vi "Graph_Get Attributes.vi"(8 "error in (no error)":errorcluster, 11 "reference in":refnum<class "Graph.lvclass">) -> (0 "error out":errorcluster, 1 "Graph DVR":refnum<data-value>, 2 "Graph Attributes":T1, 3 "reference out":refnum<class "Graph.lvclass">)   [LabVIEW 2017, in "Front Panel Publisher.lvlib" / "Graph.lvclass"]
uses:
  Graph.lvclass
  Attributes.ctl
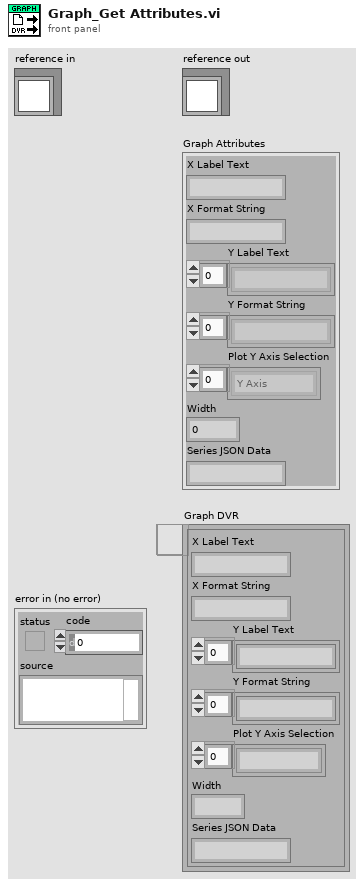
[diagram p1: front panel]
types:
  T1 = typedef "Front Panel Publisher.lvlib/Graph.lvclass/Attributes.ctl" = cluster{"X Label Text":string, "X Format String":string, "Y Label Text":string[], "Y Format String":string[], "Plot Y Axis Selection":enum16{"Y Axis", "Y2 Axis"}[], "Width":u32, "Series JSON Data":string}
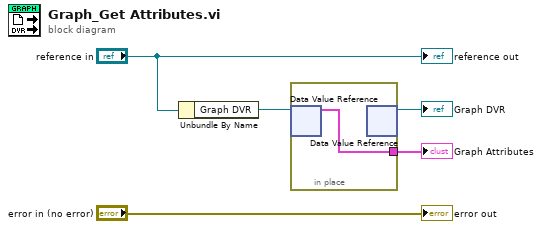
[diagram p0: block diagram]
diagram:
  n1 = Unbundle By Name("reference in") -> ("Graph DVR"=w3:refnum<data-value>)
  n2 = in-place {
    in-place-border: [w6] -> w2
    n3 = in-place-dvr #1(w3) -> (w6:T1)  [unwired: 1 out]
    n4 = in-place-dvr #1() -> (→"Graph DVR":refnum<data-value>)  [unwired: 1 in, 1 out]
  }
  "Graph Attributes" <- w2
  "error out" <- "error in (no error)"
  "reference out" <- "reference in"
